vi "Open Child.vi"(8 "error in (no error)":errorcluster, 11 "VISA Client in":refnum<class "Serial Client.lvclass">) -> (0 "error out":errorcluster, 3 "VISA Client out":refnum<class "Serial Client.lvclass">)   [LabVIEW 2020, in "Stream-Serial.lvlib" / "Serial Client.lvclass"]
uses:
  Serial Client.lvclass
  Client Command.ctl
  Stream-Serial.lvlib
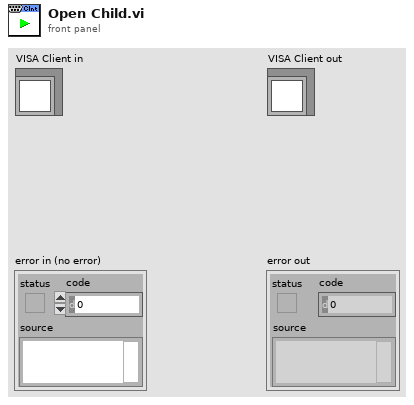
[diagram p1: front panel]
types:
  T1 = typedef "Stream-Serial.lvlib/Client Command.ctl" = enum16{"Connect", "Close", "Shutdown", "Reconnect"}
  T2 = typedef "Stream-Serial.lvlib/Serial Client.lvclass/Connection State.ctl" = enum16{"Closed", "Idle", "Connecting", "Connected", "Shutdown"}
  T3 = typedef "Stream-Serial.lvlib/Command Queue.ctl" = refnum<queue>
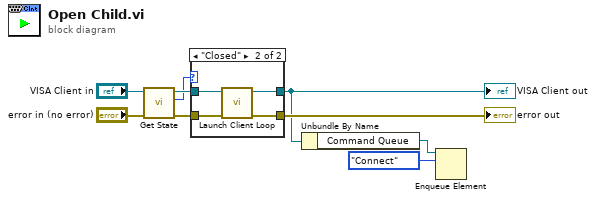
[diagram p0: block diagram]
diagram:
  n1 = call "Get State.vi"("error in (no error)"="error in (no error)", "VISA Client in"="VISA Client in") -> ("error out"=w9:errorcluster, "State"=w7:T2, "VISA Client out"=w8:refnum<class "Serial Client.lvclass">)  [unwired: 7 in]
  n2 = case shown="\"Closed\"" w7 {
    tunnel: w9 -> [w10 w14]
    tunnel: w8 -> [w11 w15]
    tunnel: [w11 w13] -> w1
    tunnel: [w10 w12] -> w4
    frame Default {
    }
    frame "Closed" {
      n3 = call "Launch Client Loop.vi"("error in (no error)"=w14, "VISA Client in"=w15) -> ("error out"=w12:errorcluster, "VISA Client out"=w13:refnum<class "Serial Client.lvclass">)  [unwired: 8 in]
    }
  }
  "error out" <- w4
  "VISA Client out" <- w1
  n4 = Unbundle By Name(w1) -> ("Command Queue"=w3:T3)
  n5 = Enqueue Element(queue=w3, element=Client_Command."Connect") -> ()  [unwired: 2 in, 3 out]
